vi "Menu.Sequeunce.Execute.vi"(8 "error in (no error)":errorcluster, 9 "Coords":T1, 10 "ItemPath":string, 11 "Cluster in":T2) -> (0 "error out":errorcluster, 3 "Cluster out":T2)   [LabVIEW 2013]
uses:
  Types/StateVariables.ctl
  Types/ChannelProperties.ctl
  <vilib>/Utility/miscctls.llb/LVPoint32TypeDef.ctl
  <vilib>/Utility/miscctls.llb/LVBoundsTypeDef.ctl
  Constants.vi
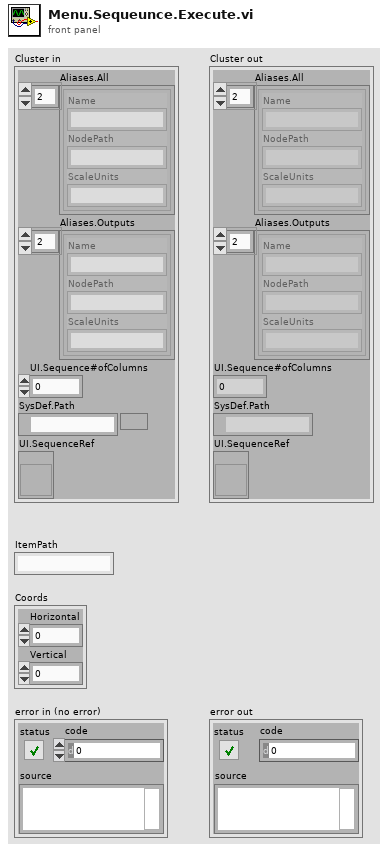
[diagram p1: front panel]
types:
  T1 = typedef "LVPoint32TypeDef.ctl" = cluster{"Horizontal":i32, "Vertical":i32}
  T2 = typedef "StateVariables.ctl" = cluster{"Aliases.All":T3[], "Aliases.Outputs":T3[], "UI.Sequence#ofColumns":i32, "SysDef.Path":path, "UI.SequenceRef":refnum<vi>}
  T3 = typedef "ChannelProperties.ctl" = cluster{"Name":string, "NodePath":string, "ScaleUnits":string}
  T4 = typedef "LVRowAndColumnTypeDef.ctl" = cluster{"Row":i32, "Column":i32}
  T5 = typedef "LVBoundsTypeDef.ctl" = cluster{"Width":u32, "Height":u32}
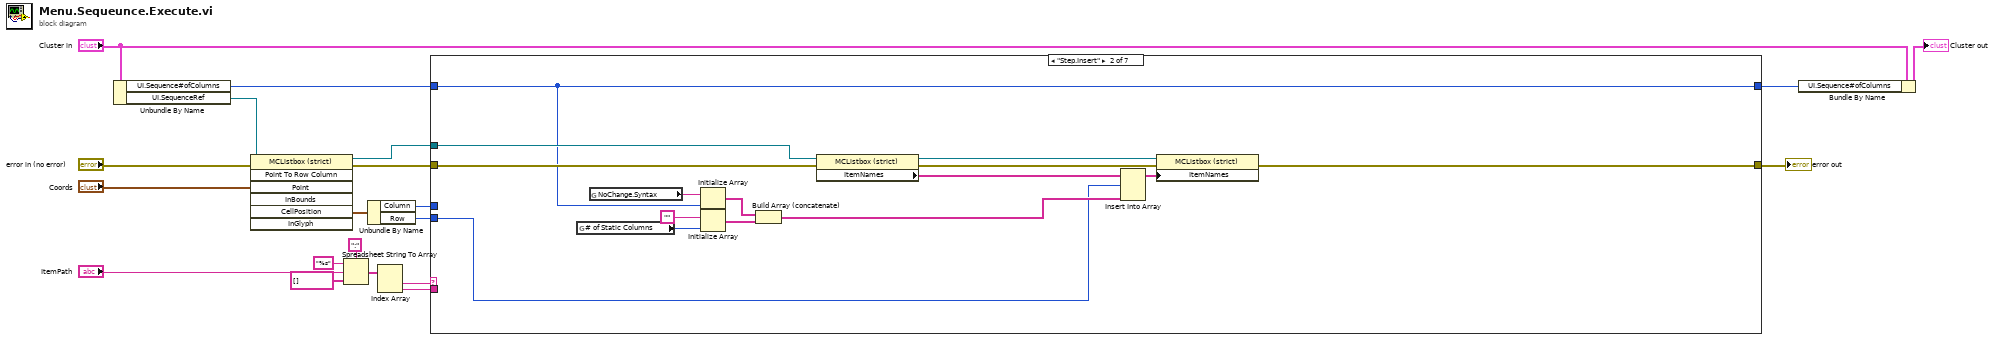
[diagram p0: block diagram]
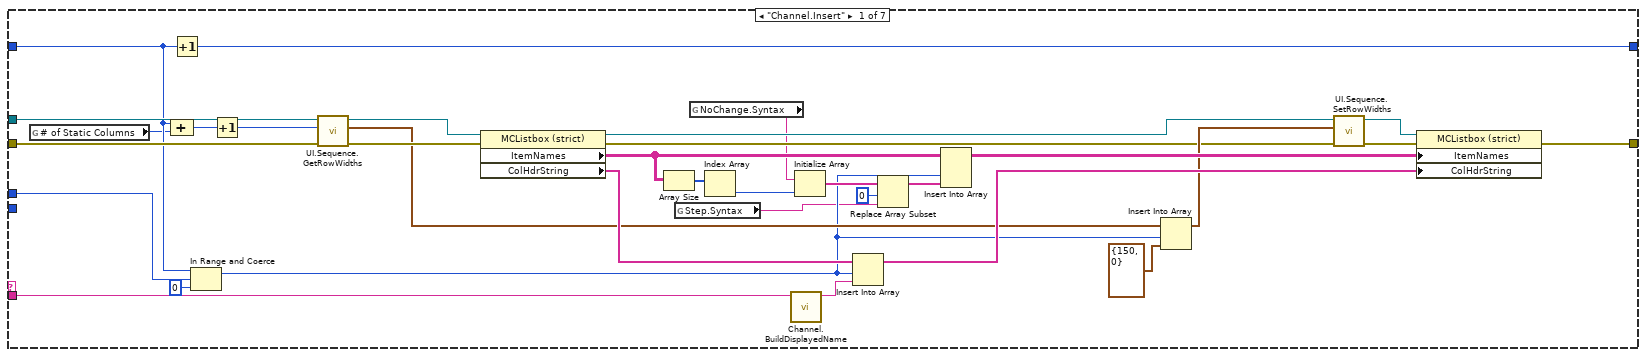
[diagram p2: hidden frame]
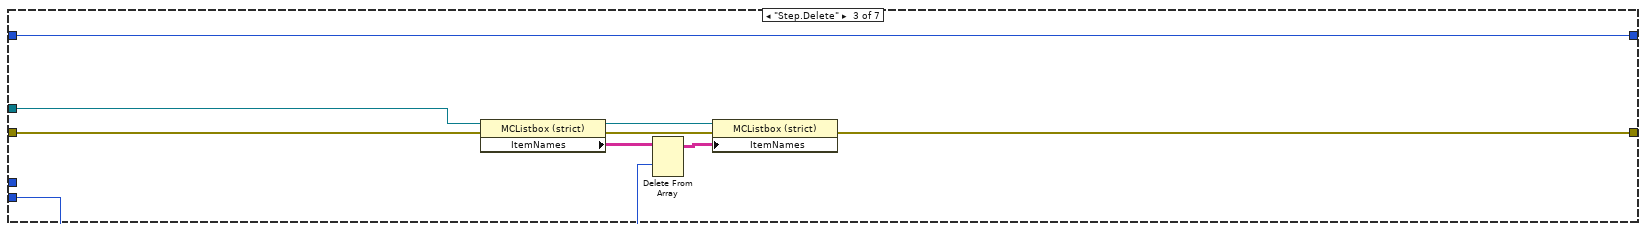
[diagram p3: hidden frame]
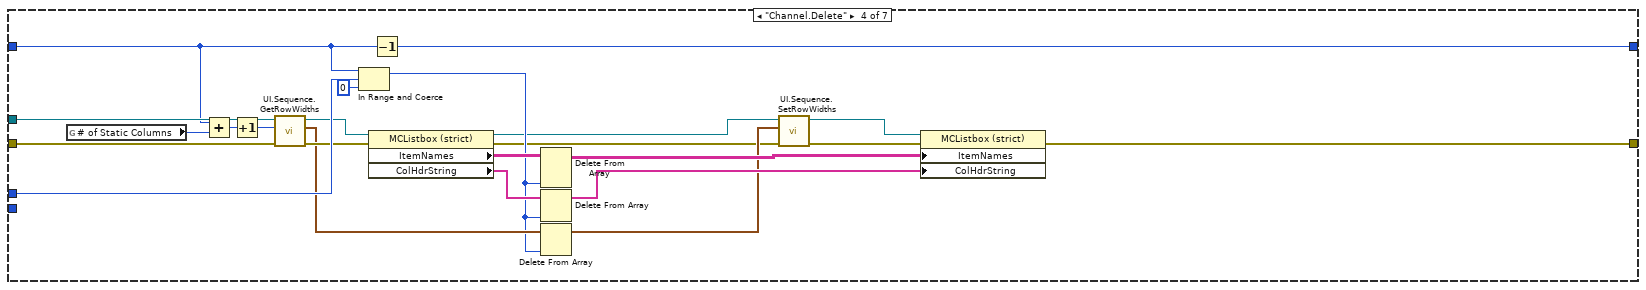
[diagram p4: hidden frame]
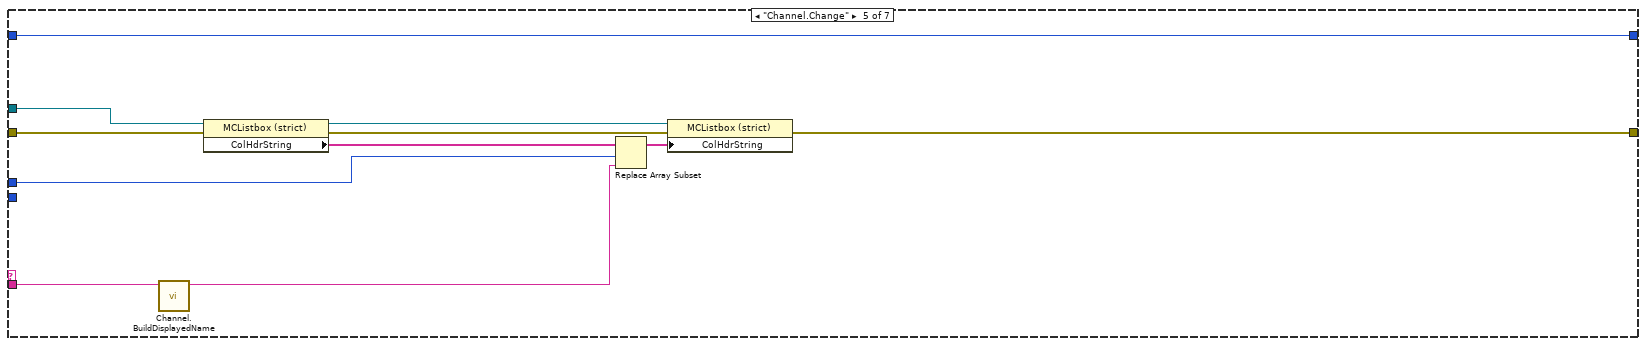
[diagram p5: hidden frame]
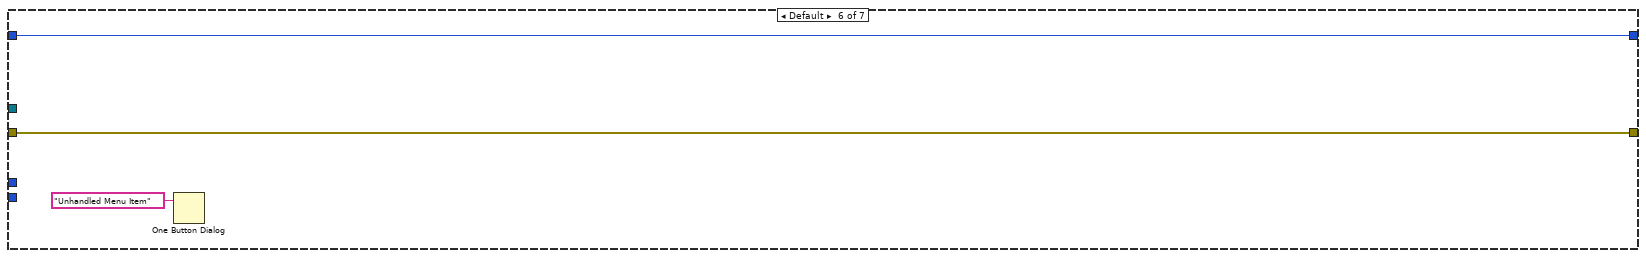
[diagram p6: hidden frame]
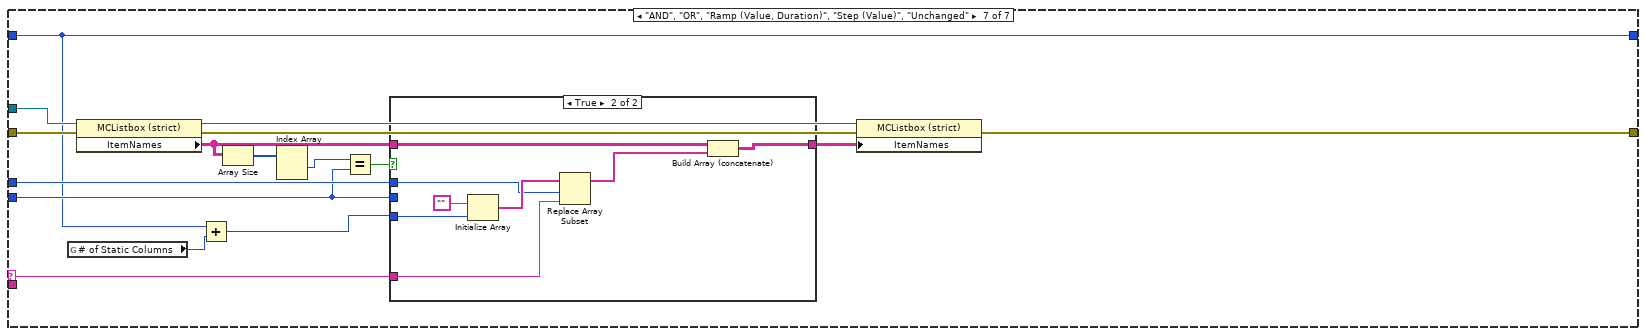
[diagram p7: hidden frame]
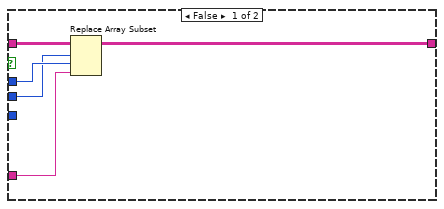
[diagram p8: hidden frame]
diagram:
  n1 = Unbundle By Name("Cluster in") -> ("UI.Sequence#ofColumns"=w11:i32, "UI.SequenceRef"=w8:refnum<vi>)
  n2 = invoke class="MCListbox (strict)" method="Point To Row Column"(reference=w8, error in="error in (no error)", "Point"="Coords") -> (reference out=w13:refnum<vi>, error out=w14:errorcluster, "CellPosition"=w10:T4)  [unwired: 4 in, 4 out]
  n3 = Spreadsheet String To Array(delimiter (Tab)=":", format string="%s", spreadsheet string="ItemPath", array type (2D Dbl)=string[] []) -> (array=w6:string[])
  n4 = Unbundle By Name(w10) -> ("Column"=w12:i32, "Row"=w1:i32)
  n5 = Index Array(array=w6) -> (element #1=w7:string, element #2=w15:string)  [unwired: 2 in]
  n6 = case shown="\"Step.Insert\"" w7 {
    selector: w7 -> [_ _ _ _ _ _ w119]
    tunnel: w11 -> [w35 w54 w69 w84 w111 w114 w117]
    tunnel: w12 -> [w53 _ _ w100 w104 _ w125]
    tunnel: w13 -> [w38 w63 w73 w91 w105 _ w129]
    tunnel: w14 -> [w40 w65 w74 w93 w106 w113 w130]
    tunnel: w15 -> [w42 _ _ _ w102 _ _]
    tunnel: [w22 w66 w75 w78 w103 w113 w118] -> w17
    tunnel: [w33 w54 w69 w98 w111 w114 w117] -> w20
    tunnel: w1 -> [_ w55 w70 _ _ _ w121]
    frame "Channel.Insert" {
      n7 = global read "Constants.vi" "# of Static Columns"() -> (w34:u32)
      n8 = Compound Arithmetic op=ADD(w35, w34) -> (w36:u32)
      n9 = Increment(x=w35) -> (x+1=w33:i32)
      n10 = In Range and Coerce(upper limit=w35, x=w53, lower limit=0) -> (coerced(x)=w30:i32)  [unwired: 1 out]
      n11 = Increment(x=w36) -> (x+1=w28:u32)
      n12 = call "UI.Sequence.GetRowWidths.vi"("error in (no error)"=w40, "Numeric"=w28, "MulticolumnListbox in"=w38) -> ("error out"=w39:errorcluster, "Array"=w31:T5[], "MulticolumnListbox out"=w37:refnum<vi>)  [unwired: 6 in]
      n13 = property class="MCListbox (strict)"(reference=w37, error in=w39) -> (reference out=w23:refnum<vi>, error out=w26:errorcluster, "ItemNames"=w50:string[][], "ColHdrString"=w45:string[])
      n14 = Array Size(array=w50) -> (size(s)=w51:i32[])
      n15 = global read "Constants.vi" "Step.Syntax"() -> (w27:string)
      n16 = global read "Constants.vi" "NoChange.Syntax"() -> (w21:string)
      n17 = Index Array(array=w51) -> (element=w49:i32)  [unwired: 1 in]
      n18 = call "Channel.BuildDisplayedName.vi"("String in"=w42) -> ("String out"=w41:string)  [unwired: 10 in]
      n19 = Initialize Array(w21, w49) -> (w48:string[])
      n20 = Insert Into Array(array=w45, index=w30, new element=w41) -> (w46:string[])
      n21 = Replace Array Subset(array=w48, new element=w27, index=0) -> (w44:string[])
      n22 = Insert Into Array(array=w50, index (col)=w30, new element=w44) -> (w47:string[][])  [unwired: 1 in]
      n23 = Insert Into Array(array=w31, index=w30, new element=T5 {"Width"=150, "Height"=0} ("new element/subarray")) -> (w32:T5[])
      n24 = call "UI.Sequence.SetRowWidths.vi"("error in (no error)"=w26, "Array"=w32, "MulticolumnListbox in"=w23) -> ("error out"=w25:errorcluster, "MulticolumnListbox out"=w24:refnum<vi>)  [unwired: 7 in]
      n25 = property class="MCListbox (strict)"(reference=w24, error in=w25, "ItemNames"=w47, "ColHdrString"=w46) -> (error out=w22:errorcluster)  [unwired: 1 out]
    }
    frame "Step.Insert" {
      n26 = global read "Constants.vi" "# of Static Columns"() -> (w62:u32)
      n27 = global read "Constants.vi" "NoChange.Syntax"() -> (w64:string)
      n28 = Initialize Array(w64, w54) -> (w59:string[])
      n29 = Initialize Array("", w62) -> (w60:string[])
      n30 = Build Array (concatenate)(w59, w60) -> (w58:string[])
      n31 = property class="MCListbox (strict)"(reference=w63, error in=w65) -> (reference out=w56:refnum<vi>, error out=w57:errorcluster, "ItemNames"=w68:string[][])
      n32 = Insert Into Array(array=w68, index (row)=w55, new element=w58) -> (w67:string[][])  [unwired: 1 in]
      n33 = property class="MCListbox (strict)"(reference=w56, error in=w57, "ItemNames"=w67) -> (error out=w66:errorcluster)  [unwired: 1 out]
    }
    frame "Step.Delete" {
      n34 = property class="MCListbox (strict)"(reference=w73, error in=w74) -> (reference out=w71:refnum<vi>, error out=w72:errorcluster, "ItemNames"=w77:string[][])
      n35 = Delete From Array(array=w77, index (row)=w70) -> (array with subset deleted=w76:string[][])  [unwired: 2 in, 1 out]
      n36 = property class="MCListbox (strict)"(reference=w71, error in=w72, "ItemNames"=w76) -> (error out=w75:errorcluster)  [unwired: 1 out]
    }
    frame "Channel.Delete" {
      n37 = global read "Constants.vi" "# of Static Columns"() -> (w86:u32)
      n38 = Add(x=w84, y=w86) -> (x+y=w85:u32)
      n39 = Increment(x=w85) -> (x+1=w83:u32)
      n40 = call "UI.Sequence.GetRowWidths.vi"("error in (no error)"=w93, "Numeric"=w83, "MulticolumnListbox in"=w91) -> ("error out"=w92:errorcluster, "Array"=w89:T5[], "MulticolumnListbox out"=w90:refnum<vi>)  [unwired: 6 in]
      n41 = In Range and Coerce(upper limit=w84, x=w100, lower limit=0) -> (coerced(x)=w88:i32)  [unwired: 1 out]
      n42 = property class="MCListbox (strict)"(reference=w90, error in=w92) -> (reference out=w79:refnum<vi>, error out=w82:errorcluster, "ItemNames"=w97:string[][], "ColHdrString"=w94:string[])
      n43 = Decrement(x=w84) -> (x-1=w98:i32)
      n44 = Delete From Array(array=w97, index (col)=w88) -> (array with subset deleted=w96:string[][])  [unwired: 2 in, 1 out]
      n45 = Delete From Array(array=w94, index=w88) -> (array with subset deleted=w95:string[])  [unwired: 1 in, 1 out]
      n46 = Delete From Array(array=w89, index=w88) -> (array with subset deleted=w87:T5[])  [unwired: 1 in, 1 out]
      n47 = call "UI.Sequence.SetRowWidths.vi"("error in (no error)"=w82, "Array"=w87, "MulticolumnListbox in"=w79) -> ("error out"=w81:errorcluster, "MulticolumnListbox out"=w80:refnum<vi>)  [unwired: 7 in]
      n48 = property class="MCListbox (strict)"(reference=w80, error in=w81, "ItemNames"=w96, "ColHdrString"=w95) -> (error out=w78:errorcluster)  [unwired: 1 out]
    }
    frame "Channel.Change" {
      n49 = call "Channel.BuildDisplayedName.vi"("String in"=w102) -> ("String out"=w101:string)  [unwired: 10 in]
      n50 = property class="MCListbox (strict)"(reference=w105, error in=w106) -> (reference out=w110:refnum<vi>, error out=w109:errorcluster, "ColHdrString"=w107:string[])
      n51 = Replace Array Subset(array=w107, new element=w101, index=w104) -> (w108:string[])
      n52 = property class="MCListbox (strict)"(reference=w110, error in=w109, "ColHdrString"=w108) -> (error out=w103:errorcluster)  [unwired: 1 out]
    }
    frame Default {
      n53 = One Button Dialog(message="Unhandled Menu Item") -> ()  [unwired: 1 in, 1 out]
    }
    frame "AND", "OR", "Ramp (Value, Duration)", "Step (Value)", "Unchanged" {
      n54 = global read "Constants.vi" "# of Static Columns"() -> (w115:u32)
      n55 = property class="MCListbox (strict)"(reference=w129, error in=w130) -> (reference out=w127:refnum<vi>, error out=w128:errorcluster, "ItemNames"=w124:string[][])
      n56 = Add(x=w117, y=w115) -> (x+y=w116:u32)
      n57 = Array Size(array=w124) -> (size(s)=w123:i32[])
      n58 = Index Array(array=w123) -> (element #1=w122:i32)  [unwired: 2 in, 1 out]
      n59 = Equal?(x=w122, y=w121) -> (x = y?=w120:bool)
      n60 = case shown="True" w120 {
        tunnel: [w135 w142] -> w126
        tunnel: w125 -> [w134 w138]
        tunnel: w124 -> [w133 w143]
        tunnel: w121 -> [w132 _]
        tunnel: w116 -> [_ w141]
        tunnel: w119 -> [w131 w137]
        frame False {
          n61 = Replace Array Subset(array=w133, new element=w131, index (row)=w132, index (col)=w134) -> (w135:string[][])
        }
        frame True {
          n62 = Initialize Array("", w141) -> (w139:string[])
          n63 = Replace Array Subset(array=w139, new element=w137, index=w138) -> (w136:string[])
          n64 = Build Array (concatenate)(w143, w136) -> (w142:string[][])
        }
      }
      n65 = property class="MCListbox (strict)"(reference=w127, error in=w128, "ItemNames"=w126) -> (error out=w118:errorcluster)  [unwired: 1 out]
    }
  }
  "error out" <- w17
  n66 = Bundle By Name(cluster="Cluster in", "UI.Sequence#ofColumns"=w20) -> (→"Cluster out":T2)
